vi "SetBase.vi"(7 "Actor":refnum<class "Actor.lvclass">, 11 "Base":T1) -> (5 "Actor":refnum<class "Actor.lvclass">)   [LabVIEW 2020, in "_Template.lvlib" / "{{Actor}}.lvlib" / "Actor.lvclass"]
uses:
  Actor.lvclass
  Actor.lvclass/Actor.ctl
  jettl/jettl/Actor/Actor.lvclass
  jettl/jettl/Lifecycle.ctl
  jettl/jettl/jettl.lvlib
  jettl/jettl/Msg/Msg.lvclass
  jettl/jettl/MsgSet.ctl
  jettl/jettl/Base.ctl
  jettl/jettl/PostSetup.ctl
  jettl/jettl/PreSetup.ctl
  jettl/jettl/Msg.ctl
  jettl/jettl/Unified.ctl
  jettl/jettl/ChildUnifiedMap.ctl
  jettl/jettl/State.ctl
panel:
  # "This front panel should not be manipulated."
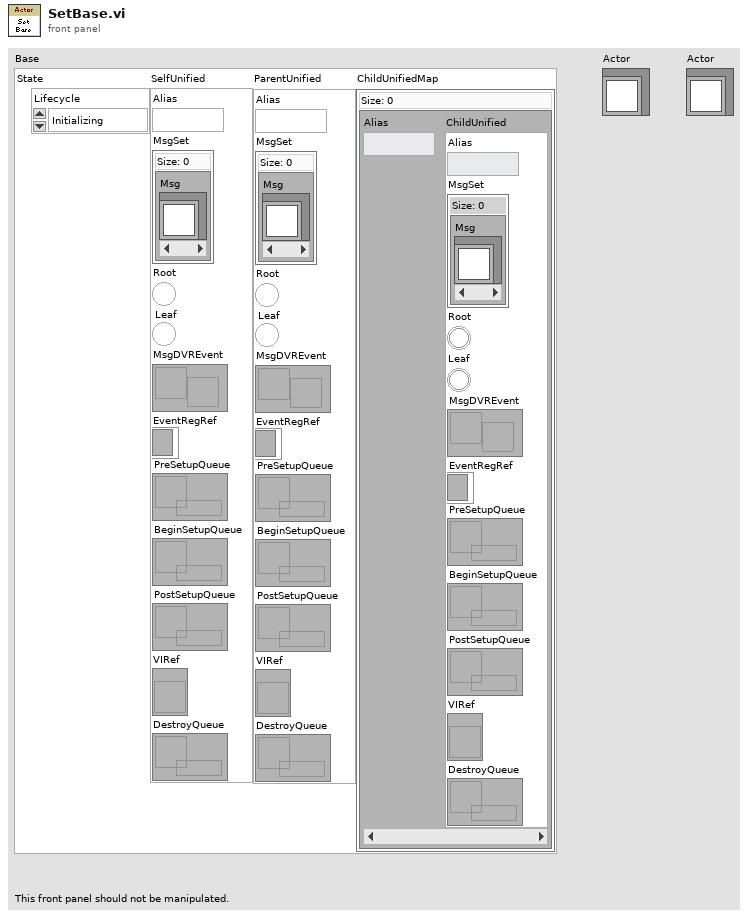
[diagram p1: front panel]
types:
  T1 = typedef "jettl.lvlib/Base.ctl" = cluster{"State":T2, "SelfUnified":T4, "ParentUnified":T4, "ChildUnifiedMap":T6}
  T2 = typedef "jettl.lvlib/State.ctl" = cluster{"Lifecycle":T3}
  T3 = typedef "jettl.lvlib/Lifecycle.ctl" = enum16{"Initializing", "SettingUp", "Starting", "Running", "Stopping", "TearingDown", "Terminated"}
  T4 = typedef "jettl.lvlib/Unified.ctl" = cluster{"Alias":string, "MsgSet":T5, "Root":bool, "Leaf":bool, "MsgDVREvent":refnum<user-event>, "EventRegRef":refnum<event-registration>, "PreSetupQueue":refnum<queue>, "BeginSetupQueue":refnum<queue>, "PostSetupQueue":refnum<queue>, "VIRef":refnum<vi>, "DestroyQueue":refnum<queue>}
  T5 = typedef "jettl.lvlib/MsgSet.ctl" = set{refnum<class "Msg.lvclass">}
  T6 = typedef "jettl.lvlib/ChildUnifiedMap.ctl" = map{string, T4}
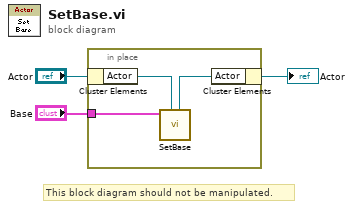
[diagram p0: block diagram]
diagram:
  # "This block diagram should not be manipulated."
  n1 = in-place {
    in-place-border: "Base" -> [w4]
    n2 = in-place-cluster #1("Actor") -> ("Actor"=w6:refnum<class "Actor.lvclass">)
    n3 = call-dynamic "SetBase.vi"("Actor"=w6, "Base"=w4) -> ("Actor"=w5:refnum<class "Actor.lvclass">)  [unwired: 9 in]
    n4 = in-place-cluster #1("Actor"=w5) -> (→"Actor":refnum<class "Actor.lvclass">)
  }
